vi "LOGGER Loop.vi"(8 "error in":errorcluster, 10 "Queues":T1, 11 "Notifiers":T2) -> (0 "error out":errorcluster)   [LabVIEW 2014, in "Logger.lvlib"]
uses:
  Logger.lvlib
  support/Message Queue/Message Queue.lvlib
  TypeDefs/Logger State.ctl
  TypeDefs/Logger Data.ctl
  Model/TypeDefs/Get Model Status Control.ctl
  Model/Model.lvlib
  <vilib>/ErrorRing/Error Ring.xnode
  <vilib>/Utility/error.llb/Error Cluster From Error Code.vi
  Support/Global names.vi
  Support/Message Queue/Message Cluster.ctl
  Support/Notifiers/Notifiers.ctl
  Support/Notifiers/Notifiers.lvlib
  Support/Message Queue/All Message Queues.ctl
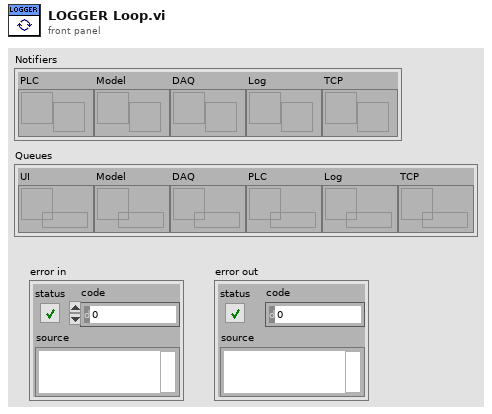
[diagram p1: front panel]
types:
  T1 = typedef "Message Queue.lvlib/All Message Queues.ctl" = cluster{"UI":refnum<queue>, "Model":refnum<queue>, "DAQ":refnum<queue>, "PLC":refnum<queue>, "Log":refnum<queue>, "TCP":refnum<queue>}
  T2 = typedef "Notifiers.lvlib/Notifiers.ctl" = cluster{"PLC":refnum<notifier>, "Model":refnum<notifier>, "DAQ":refnum<notifier>, "Log":refnum<notifier>, "TCP":refnum<notifier>}
  T3 = typedef "Logger.lvlib/Logger Data.ctl" = cluster{"tdms file out":refnum<k34>, "State":T4, "Path":path}
  T4 = typedef "Logger.lvlib/Logger State.ctl" = enum16{"Idle", "Working"}
  T5 = enum16{"open", "open or create", "create or replace", "create", "open (read-only)"}
  T6 = typedef "Model.lvlib/Get Model Status Control.ctl" = cluster{"Position":dbl, "Pump State":bool, "Fluid Flow":dbl, "Fluid Level":dbl, "Barrel Number":i32, "Spill Alarm":bool, "Level Alarm":bool}
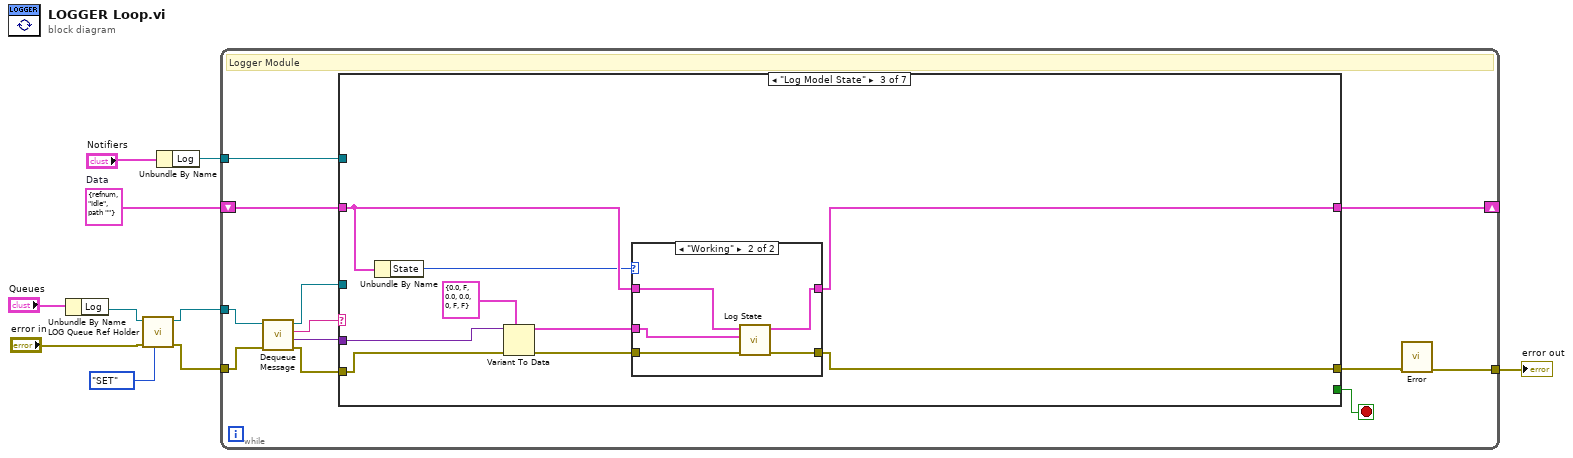
[diagram p0: block diagram]
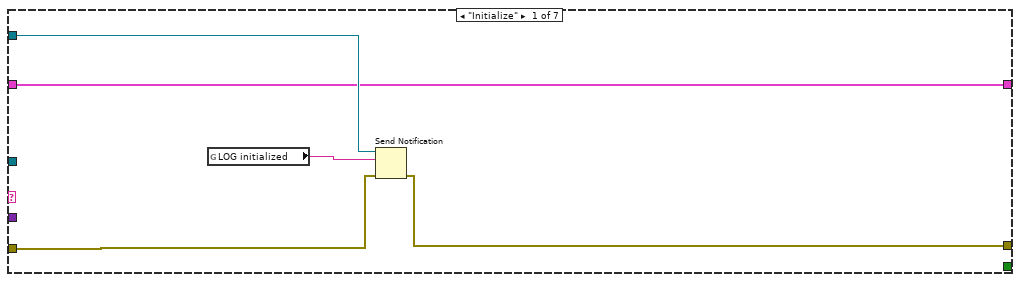
[diagram p2: hidden frame]
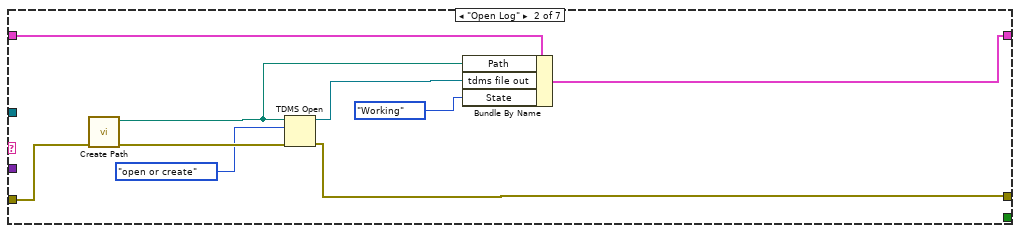
[diagram p3: hidden frame]
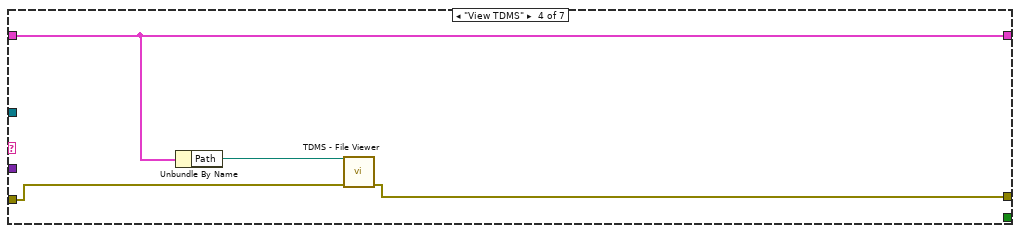
[diagram p5: hidden frame]
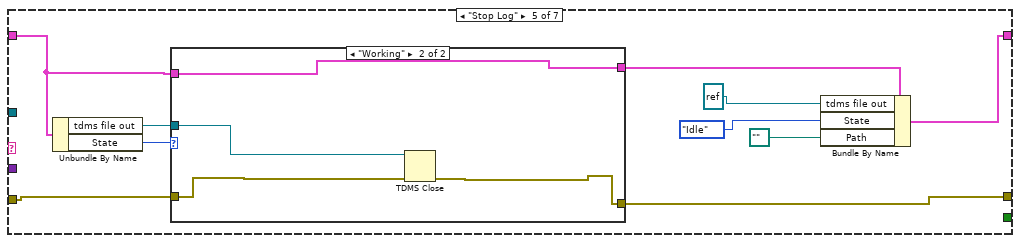
[diagram p6: hidden frame]
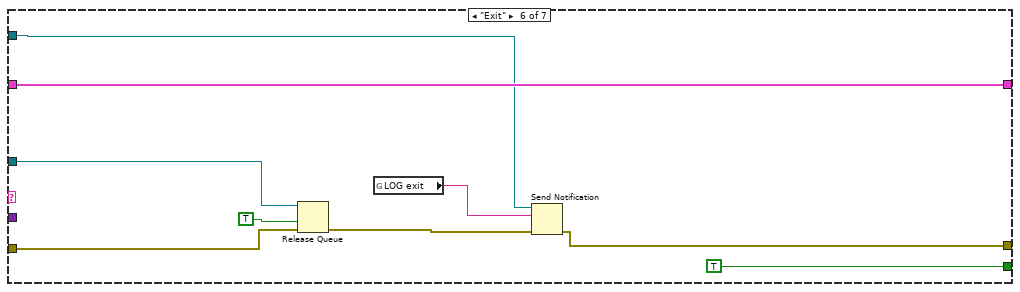
[diagram p8: hidden frame]
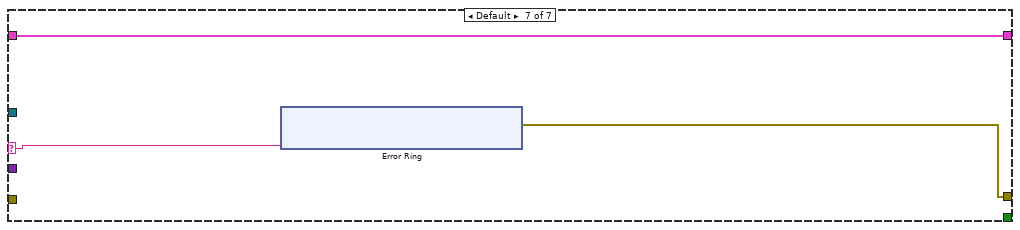
[diagram p9: hidden frame]
diagram:
  w10 = T3 {"tdms file out"=refnum, "State"=enum."Idle", "Path"=path ""}  # Data
  n1 = Unbundle By Name("Queues") -> ("Log"=w3:refnum<queue>)
  n2 = call "LOG Queue Ref Holder.vi"("Action"=enum16{"GET", "SET"}."SET", "error in"="error in", "Message Queue In"=w3) -> ("error out"=w4:errorcluster, "Input Message Queue"=w2:refnum<queue>)  [unwired: 7 in]
  n3 = Unbundle By Name("Notifiers") -> ("Log"=w6:refnum<notifier>)
  n4 = while {
    tunnel: w4 -> [w22]
    tunnel: w2 -> [w21]
    tunnel: [w11] -> w9
    shift-right: [w14] -> _
    shift-left: w10 -> [w15]
    tunnel: w6 -> [w13]
    stop <- w16 stop-if-true
    # "Logger Module"
    n5 = call "Dequeue Message.vi"("error in (no error)"=w22, "Message Queue"=w21) -> ("error out"=w20:errorcluster, "Message Data"=w17:variant, "Message"=w19:string, "dup Message Queue"=w18:refnum<queue>)  [unwired: 6 in]
    n6 = case shown="\"Log Model State\"" w19 {
      selector: w19 -> [_ _ _ _ _ _ w83]
      tunnel: w20 -> [w24 w36 w45 w56 w62 w78 _]
      tunnel: w18 -> [_ _ _ _ _ w77 _]
      tunnel: w17 -> [_ _ w43 _ _ _ _]
      tunnel: [w25 w28 w40 w54 w57 w79 w82] -> w12
      tunnel: [_ _ _ _ _ TRUE _] -> w16
      tunnel: w15 -> [w26 w33 w38 w55 w59 w81 w84]
      tunnel: [w26 w29 w39 w55 w66 w81 w84] -> w14
      tunnel: w13 -> [w27 _ _ _ _ w74 _]
      frame "Initialize" {
        n7 = global read "Global names.vi" "LOG initialized"() -> (w23:string)
        n8 = Send Notification(notification=w23, notifier=w27, error in (no error)=w24) -> (error out=w25:errorcluster)  [unwired: 1 out]
      }
      frame "Open Log" {
        n9 = call "Create Path.vi"("error in (no error)"=w36) -> ("error out"=w35:errorcluster, "File Path Control"=w31:path)  [unwired: 9 in]
        n10 = TDMS Open(8:w35, 10:T5."open or create" ("operation (0:open)"), 11:w31) -> (0:w28:errorcluster, 3:w30:refnum<k34>)  [unwired: 4 in]
        n11 = Bundle By Name(cluster=w33, "Path"=w31, "tdms file out"=w30, "State"=Logger_State."Working") -> (w29:T3)
      }
      frame "Log Model State" {
        n12 = Unbundle By Name(w38) -> ("State"=w37:T4)
        n13 = Variant To Data(error in=w45, type=T6 {"Position"=0.0, "Pump State"=FALSE, "Fluid Flow"=0.0, "Fluid Level"=0.0, "Barrel Number"=0, "Spill Alarm"=FALSE, "Level Alarm"=FALSE} ("Model Status"), Variant=w43) -> (data=w42:T6, error out=w41:errorcluster)
        n14 = case shown="\"Working\"" w37 {
          tunnel: w42 -> [_ w52]
          tunnel: w41 -> [w46 w51]
          tunnel: [w46 w48] -> w40
          tunnel: [w47 w49] -> w39
          tunnel: w38 -> [w47 w50]
          frame Default {
          }
          frame "Working" {
            n15 = call "Log State.vi"("error in (no error)"=w51, "Model Status"=w52, "Data"=w50) -> ("error out"=w48:errorcluster, "Data out"=w49:T3)  [unwired: 7 in]
          }
        }
      }
      frame "View TDMS" {
        n16 = Unbundle By Name(w55) -> ("Path"=w53:path)
        n17 = call <vilib>:"TDMS - File Viewer.vi"("error in (no error)"=w56, "file path"=w53) -> ("error out"=w54:errorcluster)  [unwired: 4 in, 1 out]
      }
      frame "Stop Log" {
        n18 = Unbundle By Name(w59) -> ("tdms file out"=w63:refnum<k34>, "State"=w60:T4)
        n19 = case shown="\"Working\"" w60 {
          tunnel: w63 -> [_ w69]
          tunnel: w62 -> [w68 w70]
          tunnel: [w68 w71] -> w57
          tunnel: w59 -> [w67 w72]
          tunnel: [w67 w72] -> w58
          frame "Idle", Default {
          }
          frame "Working" {
            n20 = TDMS Close(8:w70, 11:w69) -> (0:w71:errorcluster)  [unwired: 1 out]
          }
        }
        n21 = Bundle By Name(cluster=w58, "tdms file out"=refnum<k34> refnum, "State"=Logger_State."Idle", "Path"=path "") -> (w66:T3)
      }
      frame "Exit" {
        n22 = Release Queue(queue=w77, force destroy? (F)=TRUE, error in (no error)=w78) -> (error out=w76:errorcluster)  [unwired: 2 out]
        n23 = global read "Global names.vi" "LOG exit"() -> (w73:string)
        n24 = Send Notification(notification=w73, notifier=w74, error in (no error)=w76) -> (error out=w79:errorcluster)  [unwired: 1 out]
      }
      frame Default {
        n25 = xnode "Error Ring"("parameter 0"=w83) -> ("error out"=w82:errorcluster)
      }
    }
    n26 = call "Error.vi"("error in"=w12) -> ("error out"=w11:errorcluster)  [unwired: 10 in]
  }
  "error out" <- w9
